vi "pid_loop.vi"(0 "Current Pos":dbl, 5 "Desired Pos":dbl, 7 "P":dbl, 9 "I":dbl, 11 "D":dbl, 12 "dt":dbl, 13 "Update PID (F)":bool) -> (4 "Voltage Output":dbl)   [LabVIEW 2011]
doc: "Standard PID loop. \nSee: http://en.wikipedia.org/wiki/PID_controller"
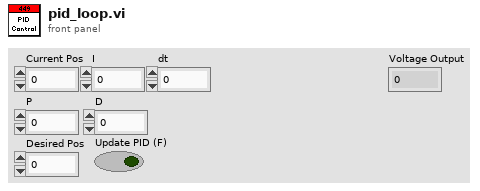
[diagram p1: front panel]
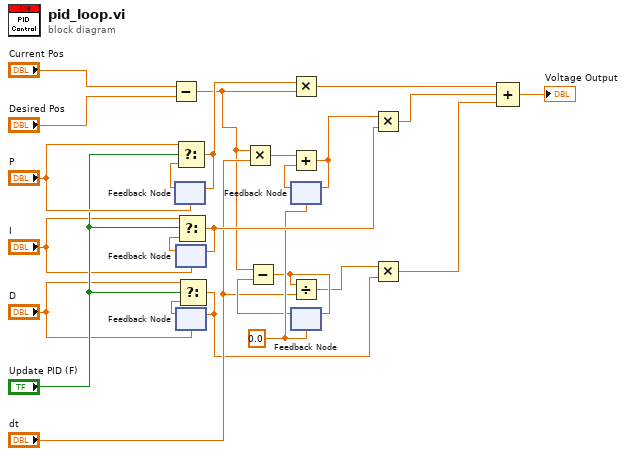
[diagram p0: block diagram]
diagram:
  w10 = 0.0
  n1 = Subtract(x="Current Pos", y="Desired Pos") -> (x-y=w1:dbl)
  n2 = feedback #1("P") -> (w24:dbl)
  n3 = Select(t="P", s="Update PID (F)", f=w24) -> (s? t:f=w15:dbl)
  n4 = feedback-in #1(w15) -> ()
  n5 = feedback #2("I") -> (w21:dbl)
  n6 = feedback #3("D") -> (w22:dbl)
  n7 = Select(t="I", s="Update PID (F)", f=w21) -> (s? t:f=w12:dbl)
  n8 = feedback-in #2(w12) -> ()
  n9 = Select(t="D", s="Update PID (F)", f=w22) -> (s? t:f=w3:dbl)
  n10 = feedback-in #3(w3) -> ()
  n11 = Multiply(x=w1, y="dt") -> (x*y=w9:dbl)
  n12 = Multiply(x=w15, y=w1) -> (x*y=w16:dbl)
  n13 = feedback #4(w10) -> (w14:dbl)
  n14 = Add(x=w9, y=w14) -> (x+y=w13:dbl)
  n15 = feedback-in #4(w13) -> ()
  n16 = feedback #5(w10) -> (w7:dbl)
  n17 = Subtract(x=w1, y=w7) -> (x-y=w6:dbl)
  n18 = Divide(x=w6, y="dt") -> (x/y=w4:dbl)
  n19 = feedback-in #5(w6) -> ()
  n20 = Multiply(x=w13, y=w12) -> (x*y=w11:dbl)
  n21 = Multiply(x=w4, y=w3) -> (x*y=w2:dbl)
  n22 = Compound Arithmetic op=ADD(w16, w11, w2) -> (→"Voltage Output":dbl)
